vi "DaqInit.vi"() -> (0 "error out":errorcluster, 3 "Refnum out":refnum<k21>)   [LabVIEW 2020]
uses:
  <vilib>/DAQmx/create/channels.llb/DAQmx Create Channel (AI-Voltage-Custom with Excitation).vi
  <vilib>/DAQmx/configure/timing.llb/DAQmx Timing (Sample Clock).vi
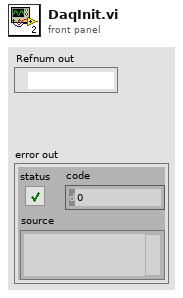
[diagram p1: front panel]
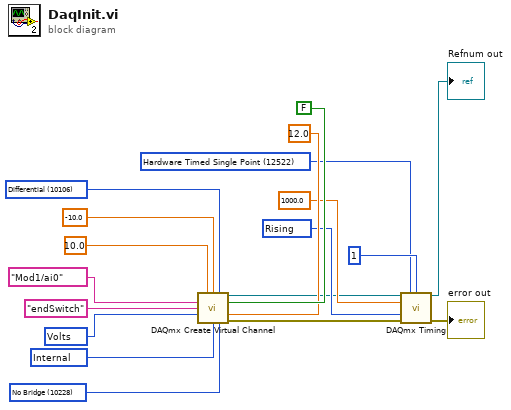
[diagram p0: block diagram]
diagram:
  w6 = 10280 items=["Rising"=10280, "Falling"=10171] ("active edge")
  w3 = 12522 items=["Finite Samples"=10178, "Continuous Samples"=10123, "Hardware Timed Single Point"=12522] ("sample mode")
  w15 = 10228 items=["Full Bridge"=10182, "Half Bridge"=10187, "Quarter Bridge"=10270, "No Bridge"=10228] ("bridge configuration")
  w14 = 10200 items=["Internal"=10200, "External"=10167, "None"=10230] ("voltage excitation source")
  w12 = 10348 items=["Volts"=10348, "From Custom Scale"=10065] ("units")
  w9 = 10106 items=["Default"=-1, "RSE"=10083, "NRSE"=10078, "Differential"=10106, "Pseudodifferential"=12529] ("input terminal configuration")
  n1 = call-poly <vilib>:"DAQmx Create Virtual Channel.vi"("maximum value"=10.0, "minimum value"=-10.0, "input terminal configuration"=w9, "physical channels"=tag "Mod1/ai0", "use excitation for scaling"=FALSE, "name to assign"="endSwitch", "units"=w12, "voltage excitation value"=12.0, "voltage excitation source"=w14, "bridge configuration"=w15) -> ("task out"=w1:refnum<k21>, "error out"=w2:errorcluster)  [unwired: 4 in]
  n2 = call-poly <vilib>:"DAQmx Timing.vi"("task/channels in"=w1, "sample mode"=w3, "samples per channel"=1, "rate"=1000.0, "active edge"=w6, "error in"=w2) -> ("task out"=→"Refnum out":refnum<k21>, "error out"=→"error out":errorcluster)  [unwired: 8 in]
